vi "Hypertext Link Anchor.vi"(0 "Leading":sgl=1.5, 1 "Text zone (points)":cluster{"widht":sgl, "height":sgl}={"widht"=612.0, "height"=792.0}, 3 "Image offsetY":sgl, 5 "Hyperlink":T3, 7 "Image to Add refnum [ ]":T2, 9 "Font refnum":refnum<k24>, 11 "error in (no error)":errorcluster, 13 "Paragraph indentation (points)":T1) -> (4 "Leading OUT":sgl=1.5, 6 "Anchor":refnum<k24>, 15 "error out":errorcluster)   [LabVIEW 2012]
doc: "Creates a <B>text hyperlink</B>.\n\nVersion 1.0\nDeveloped by Jean-Marc Simard\nCopyright © 2010, Exaprom Inc.\nAll rights reserved.\nLicense: BSD\n\nWith iTextSharp 4.1.6 (http://itextsharp.sourceforge.net)\nunder Mozilla Public License Version 1.1\n(http://www.mozilla.org/MPL/MPL-1.1.html)"
uses:
  Controls/Text and Hypertext.ctl
  C:/Users/MaxCorp/Documents/TopPerm - Base/DLL/itextsharp.dll
  DLL/itextsharp.dll
  Controls/Image to Add refnum [ ].ctl
  Controls/Paragraph indentation.ctl
  Controls/Phrase or paragraph.ctl
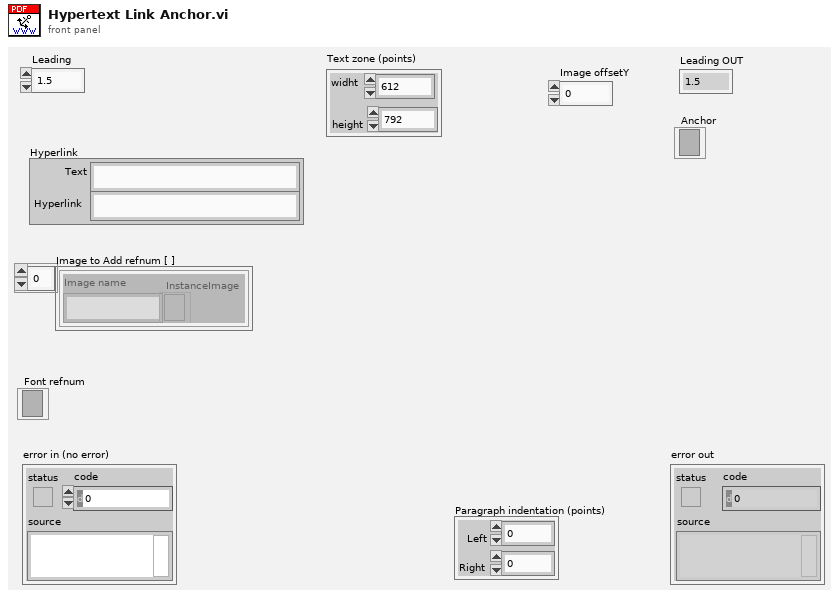
[diagram p1: front panel]
types:
  T1 = typedef "Paragraph indentation.ctl" = cluster{"Left":sgl, "Right":sgl}
  T2 = typedef "Image to Add refnum [ ].ctl" = cluster{"Image name":string, "InstanceImage":refnum<k24>}[]
  T3 = typedef "Text and Hypertext.ctl" = cluster{"Text":string, "Hyperlink":string}
  T4 = typedef "Phrase or paragraph.ctl" = enum16{"Add to Phrase", "Add to Paragraph", "Create Phrase", "Create Paragraph"}
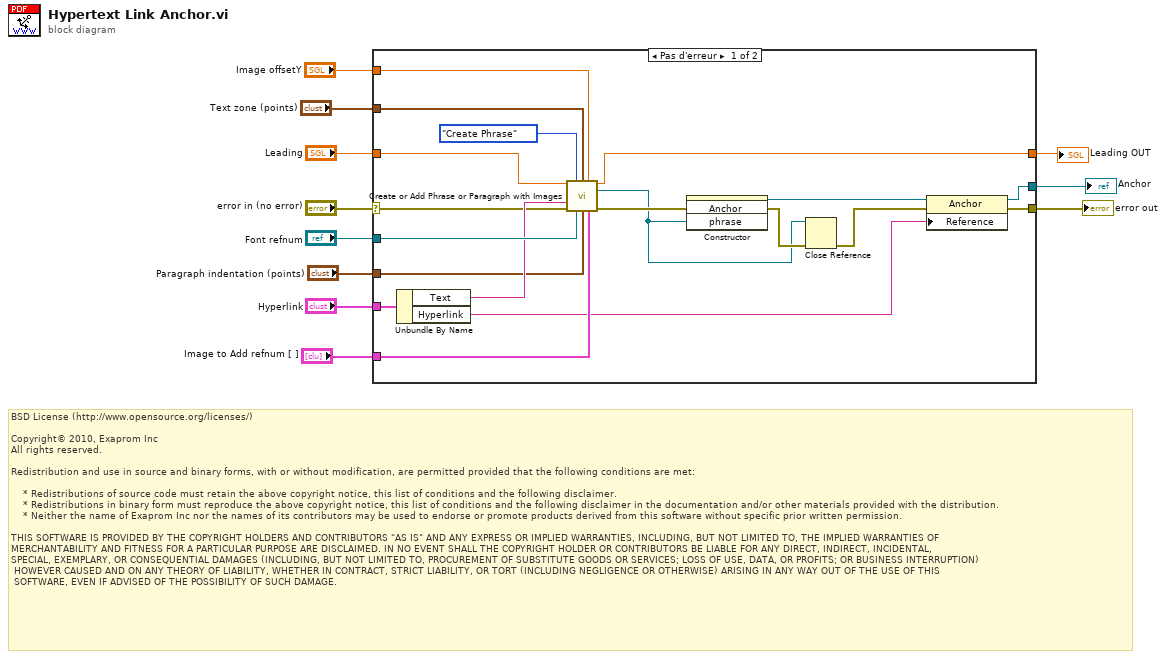
[diagram p0: block diagram]
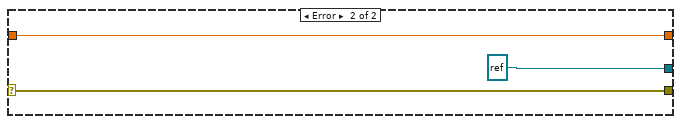
[diagram p2: hidden frame]
diagram:
  # "BSD License (http://www.opensource.org/licenses/)\n\nCopyright© 2010, Exaprom Inc\nAll rights reserved.\n\nRedistribution and use in source and binary forms, with or without modification, are permitted provided that the following conditions are met:\n\n    * Redistributions of source code must retain the above copyright notice, this list of conditions and the following disclaimer.\n    * Redistributions in binary form must reproduce the above copyright notice, this list of conditions and the following disclaimer in the documentation and/or other materials provided with the distribution.\n    * Neither the name of Exaprom Inc nor the names of its contributors may be used to endorse or promote products derived from this software without specific prior written permission.\n\nTHIS SOFTWARE IS PROVIDED BY THE COPYRIGHT HOLDERS AND CONTRIBUTORS \"AS IS\" AND ANY EXPRESS OR IMPLIED WARRANTIES, INCLUDING, BUT NOT LIMITED TO, THE IMPLIED WARRANTIES OF \nMERCHANTABILITY AND FITNESS FOR A PARTICULAR PURPOSE ARE DISCLAIMED. IN NO EVENT SHALL THE COPYRIGHT HOLDER OR CONTRIBUTORS BE LIABLE FOR ANY DIRECT, INDIRECT, INCIDENTAL,\nSPECIAL, EXEMPLARY, OR CONSEQUENTIAL DAMAGES (INCLUDING, BUT NOT LIMITED TO, PROCUREMENT OF SUBSTITUTE GOODS OR SERVICES; LOSS OF USE, DATA, OR PROFITS; OR BUSINESS INTERRUPTION)\n HOWEVER CAUSED AND ON ANY THEORY OF LIABILITY, WHETHER IN CONTRACT, STRICT LIABILITY, OR TORT (INCLUDING NEGLIGENCE OR OTHERWISE) ARISING IN ANY WAY OUT OF THE USE OF THIS\n SOFTWARE, EVEN IF ADVISED OF THE POSSIBILITY OF SUCH DAMAGE."
  n1 = case shown="Pas d'erreur" "error in (no error)" {
    selector: "error in (no error)" -> [w14 w33]
    tunnel: [w26 w33] -> w11
    tunnel: "Hyperlink" -> [w29 _]
    tunnel: [w25 refnum<k24> refnum ("hidden reference")] -> w8
    tunnel: "Leading" -> [w16 w31]
    tunnel: "Font refnum" -> [w24 _]
    tunnel: "Image to Add refnum [ ]" -> [w30 _]
    tunnel: "Text zone (points)" -> [w23 _]
    tunnel: "Paragraph indentation (points)" -> [w17 _]
    tunnel: [w15 w31] -> w3
    tunnel: "Image offsetY" -> [w13 _]
    frame No Error {
      n2 = Unbundle By Name(w29) -> ("Text"=w21:string, "Hyperlink"=w28:string)
      n3 = call "Create or Add Phrase or Paragraph with Images.vi"("Leading"=w16, "Phrase or paragraph"=Phrase_or_paragraph."Create Phrase", "Text zone (points)"=w23, "Image offsetY"=w13, "Text"=w21, "error in (no error)"=w14, "Font refnum"=w24, "Paragraph indentation (points)"=w17, "Image to Add refnum [ ]"=w30) -> ("Leading duplicate"=w15:sgl, "Phrase refnum OUT"=w18:refnum<k24>, "error out"=w22:errorcluster)  [unwired: 2 in, 2 out]
      n4 = constructor class="Anchor"(error in=w22, "phrase"=w18) -> (reference out=w27:refnum<k24>, error out=w20:errorcluster)  [unwired: 2 in, 2 out]
      n5 = Close Reference(reference=w18, error in (no error)=w20) -> (error out=w19:errorcluster)
      n6 = property class="Anchor"(reference=w27, error in=w19, "Reference"=w28) -> (reference out=w25:refnum<k24>, error out=w26:errorcluster)
    }
    frame Error {
    }
  }
  "error out" <- w11
  "Anchor" <- w8
  "Leading OUT" <- w3
